vi "getFilterWheelPosition.vi"(6 "Delay between send and receive [ms]":i32=100, 8 "error in (no error)":errorcluster, 10 "locationId":i32, 11 "Monochromator in":refnum<class "Monochromator.lvclass">) -> (0 "error out":errorcluster, 2 "position":i32, 3 "Monochromator out":refnum<class "Monochromator.lvclass">)   [LabVIEW 2020, in "horiba.lvlib" / "Monochromator.lvclass"]
doc: "Returns the current filter wheel position.\n\nparameter description\nindex Integer. Used to identify which mono to control. See mono_list command\nlocationId Integer. Specifies the filter wheel location.\n1 = Filter wheel 1 (Internal)\n2 = Filter wheel 2 (External)"
uses:
  Monochromator.lvclass
  FilterWheelPosition.ctl
  f4fe725d-34e7-4b43-af30-976d270c3ce5.vi
  d9b87029-586e-44ee-a6e5-d4a5e0edce38.vi
  b59fd1e7-dcda-425c-bd6c-61aafb79e7f4.vi
  <vilib>/JDP Science/JSONtext/Variant to JSON Text.vi
  <vilib>/JDP Science/JSONtext/Set Item.vi
  <vilib>/JDP Science/JSONtext/JSON text to Variant.vi
  <vilib>/JDP Science/JSONtext/LVClass Serializer/JSONtext LVClass Serializer.lvclass
  GenericDevice/GenericDevice.lvclass
panel:
  # "Connector Pane"
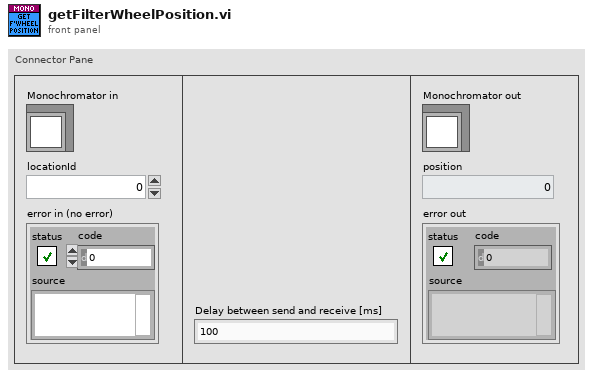
[diagram p1: front panel]
types:
  T1 = typedef "horiba.lvlib/Monochromator.lvclass/FilterWheelPosition.ctl" = cluster{"position":i32}
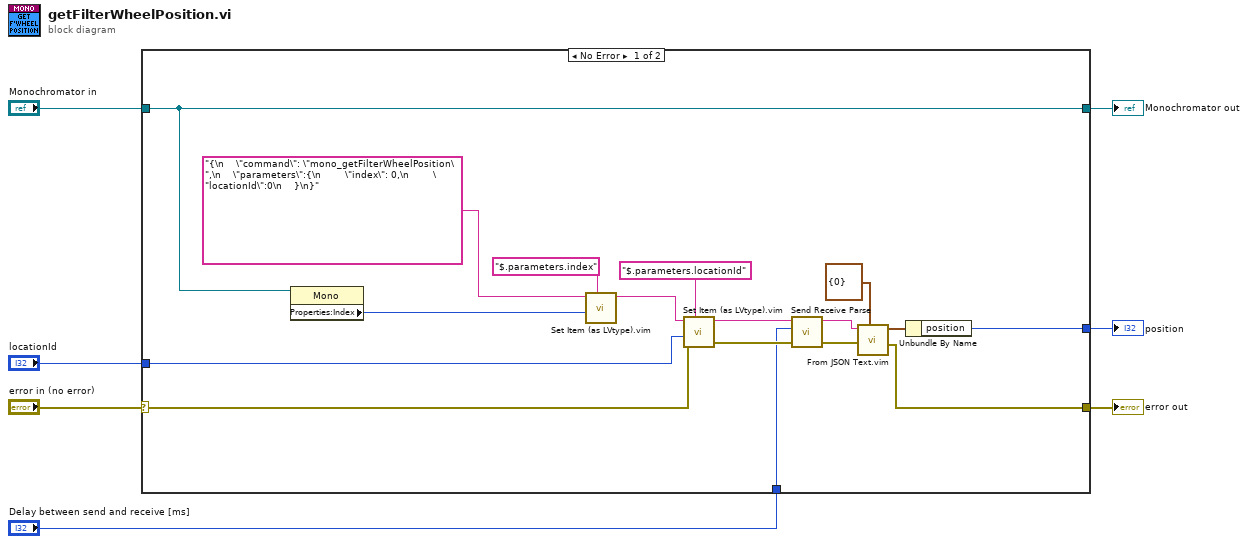
[diagram p0: block diagram]
diagram:
  n1 = case shown="No Error" "error in (no error)" {
    selector: "error in (no error)" -> [w23 w26]
    tunnel: [w22 w26] -> w6
    tunnel: [w13 w25] -> w4
    tunnel: "Monochromator in" -> [w13 w25]
    tunnel: [w16 _] -> w3
    tunnel: "Delay between send and receive [ms]" -> [w14 _]
    tunnel: "locationId" -> [w8 _]
    frame No Error {
      n2 = property class="Mono"(reference=w13) -> ("Properties:Index"=w10:i32)  [unwired: 1 in, 2 out]
      n3 = call "Set Item (as LVtype).vim"("$Path or Item Name"="$.parameters.index", "Anything"=w10, "JSON"="{\n    \"command\": \"mono_getFilterWheelPosition\",\n    \"parameters\":{\n        \"index\": 0,\n        \"locationId\":0\n    }\n}") -> ("<JSON>"=w12:string)  [unwired: 5 in, 2 out]
      n4 = call "Set Item (as LVtype).vim"("$Path or Item Name"="$.parameters.locationId", "error in (no error)"=w23, "Anything"=w8, "JSON"=w12) -> ("error out"=w21:errorcluster, "<JSON>"=w18:string)  [unwired: 4 in, 1 out]
      n5 = call "Send Receive Parse.vi"("error in"=w21, "Delay between send and receive [ms]"=w14, "<JSON>"=w18) -> ("error out"=w19:errorcluster, "results-JSON string"=w20:string)  [unwired: 6 in, 1 out]
      n6 = call "From JSON Text.vim"("Data Type and Default Value"=T1 {"position"=0} ("Wavelength Position"), "error in (no error)"=w19, "JSON"=w20) -> ("error out"=w22:errorcluster, "Data out"=w17:T1)  [unwired: 7 in]
      n7 = Unbundle By Name(w17) -> ("position"=w16:i32)
    }
    frame Error {
    }
  }
  "error out" <- w6
  "Monochromator out" <- w4
  "position" <- w3
